vi "Parse Power Level.vi"(8 "error in":errorcluster, 10 "Read Values":string[](array[string]), 11 "2936r in":refnum<class "2936r.lvclass">) -> (0 "error out":errorcluster, 2 "Power (W)":dbl[](array[numeric]), 3 "2936r out":refnum<class "2936r.lvclass">)   [LabVIEW 2018, in "2936r.lvlib" / "2936r.lvclass"]
uses:
  2936r.lvclass
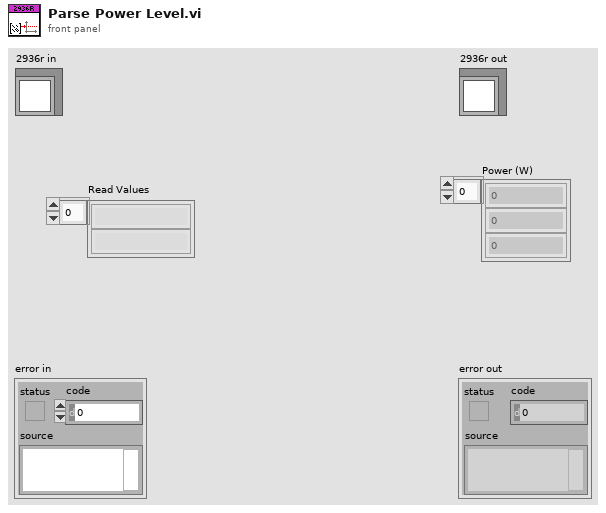
[diagram p1: front panel]
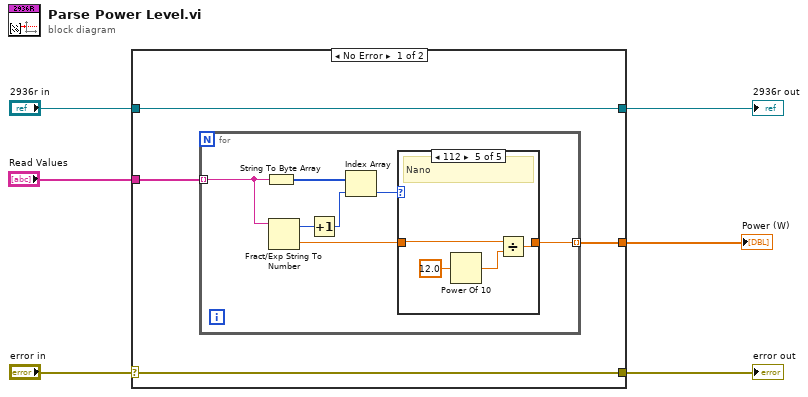
[diagram p0: block diagram]
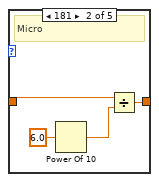
[diagram p3: hidden frame]
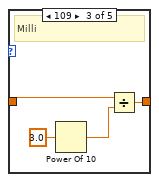
[diagram p4: hidden frame]
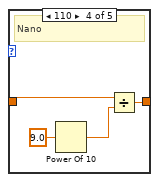
[diagram p5: hidden frame]
diagram:
  n1 = case shown="No Error" "error in" {
    selector: "error in" -> [w10 w36]
    tunnel: [w10 w36] -> w5
    tunnel: [w9 w35] -> w3
    tunnel: "2936r in" -> [w9 w35]
    tunnel: "Read Values" -> [w8 _]
    tunnel: [w7 _] -> w1
    frame No Error {
      n2 = for {
        tunnel: w8 -> [w17] mode=indexing
        tunnel: [w11] -> w7 mode=indexing
        n3 = String To Byte Array(string=w17) -> (unsigned byte array=w15:u8[])
        n4 = Fract/Exp String To Number(string=w17) -> (offset past number=w16:i32, number=w12:dbl)  [unwired: 3 in]
        n5 = Increment(x=w16) -> (x+1=w14:i32)
        n6 = Index Array(array=w15, index=w14) -> (element=w13:u8)
        n7 = case shown="112" w13 {
          tunnel: w12 -> [w18 w22 w26 w30 w34]
          tunnel: [w18 w21 w25 w29 w33] -> w11
          frame 0, Default {
          }
          frame 181 {
            # "Micro"
            n8 = Power Of 10(x=6.0) -> (10^x=w19:dbl)
            n9 = Divide(x=w22, y=w19) -> (x/y=w21:dbl)
          }
          frame 109 {
            # "Milli"
            n10 = Power Of 10(x=3.0) -> (10^x=w23:dbl)
            n11 = Divide(x=w26, y=w23) -> (x/y=w25:dbl)
          }
          frame 110 {
            # "Nano"
            n12 = Power Of 10(x=9.0) -> (10^x=w27:dbl)
            n13 = Divide(x=w30, y=w27) -> (x/y=w29:dbl)
          }
          frame 112 {
            # "Nano"
            n14 = Power Of 10(x=12.0) -> (10^x=w31:dbl)
            n15 = Divide(x=w34, y=w31) -> (x/y=w33:dbl)
          }
        }
      }
    }
    frame Error {
    }
  }
  "error out" <- w5
  "2936r out" <- w3
  "Power (W)" <- w1
